vi "Receive Results Object.vi"(8 "error in (no error)":errorcluster, 10 "Results.lvclass":refnum<class "Results.lvclass">, 11 "Client Controller in":refnum<class "Client Controller.lvclass">) -> (0 "error out":errorcluster, 3 "Client Controller out":refnum<class "Client Controller.lvclass">)   [LabVIEW 2026, in "Client Controller.lvlib" / "Client Controller.lvclass"]
uses:
  Client Controller.lvclass
  MAL-Framework/user.lib/Common Components/Results/Results.lvclass
  MAL-Framework/user.lib/Common Components/Controller/Messages/Send Results Object/Send Results Object.lvclass
  C:/Program Files/National Instruments/LabVIEW 2026/vi.lib/ActorFramework/Message/Message.lvclass
  Client Controller.lvclass/Client Controller.ctl
  MAL-Framework/user.lib/Common Components/Controller/Controller.lvclass
  <vilib>/ActorFramework/Message Enqueuer/Message Enqueuer.lvclass
  recovery/packages/ni_lib_linked_network_actor-1.2.0.19-9492AF5A82/File Group 0/vi.lib/NI/Actors/Linked Network Actor/Linked Network Actor Messages/Transmit Network Message Msg/Transmit Network Message Msg.lvclass
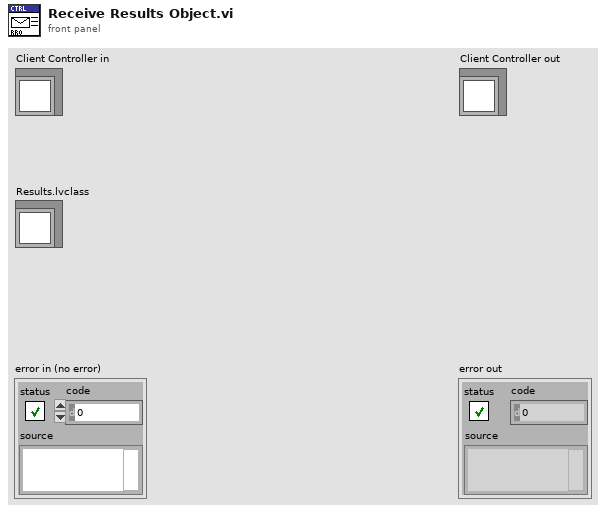
[diagram p1: front panel]
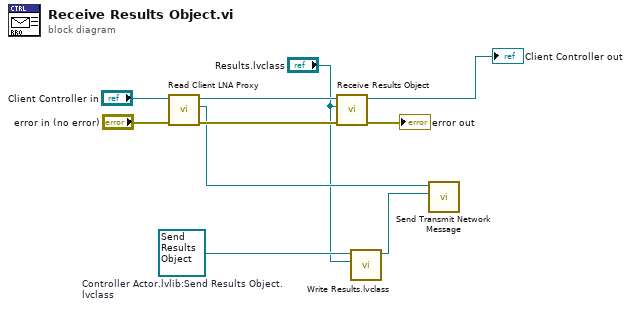
[diagram p0: block diagram]
diagram:
  w3 = refnum<class "Send Results Object.lvclass"> refnum  # Controller Actor.lvlib:Send Results Object.lvclass
  n1 = call "Read Client LNA Proxy.vi"("error in (no error)"="error in (no error)", "Client Controller in"="Client Controller in") -> ("error out"=w6:errorcluster, "Actor Framework:Message Enqueuer"=w4:refnum<class "Message Enqueuer.lvclass">, "Client Controller out"=w8:refnum<class "Client Controller.lvclass">)  [unwired: 7 in]
  n2 = call-parent "Receive Results Object.vi"("error in (no error)"=w6, "Results.lvclass"="Results.lvclass", "Controller in"=w8) -> ("error out"=→"error out":errorcluster, "Controller out"=→"Client Controller out":refnum<class "Client Controller.lvclass">)  [unwired: 7 in]
  n3 = call "Write Results.lvclass.vi"("Results.lvclass"="Results.lvclass", "Send Results Object in"=w3) -> ("Send Results Object out"=w1:refnum<class "Send Results Object.lvclass">)  [unwired: 8 in, 1 out]
  n4 = call "Send Transmit Network Message.vi"("Message"=w1, "Message Enqueuer"=w4) -> ()  [unwired: 8 in, 2 out]
